vi "tt_timeandsamples.vi"(6 "bin":dbl, 9 "refreshtime":dbl, 10 "srateAODOtt":dbl, 11 "tot#ofsamples":i32) -> (1 "refreshrate":dbl, 2 "refreshbuffer":i32, 3 "timetracecycles":i32)   [LabVIEW 2015]
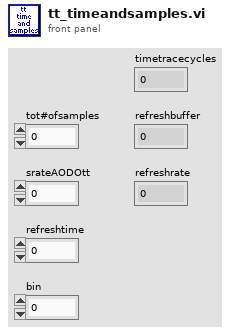
[diagram p1: front panel]
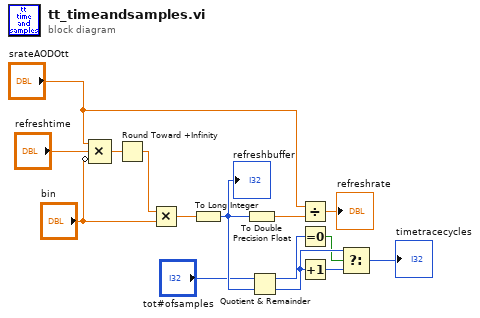
[diagram p0: block diagram]
diagram:
  n1 = Compound Arithmetic op=MULTIPLY("srateAODOtt", "refreshtime", invert "bin") -> (w2:dbl)
  n2 = Round Toward +Infinity(x=w2) -> (ceil(x): smallest int >= x=w9:dbl)
  n3 = Multiply(x=w9, y="bin") -> (x*y=w10:dbl)
  n4 = To Long Integer(number=w10) -> (32bit integer=w12:i32)
  "refreshbuffer" <- w12
  n5 = To Double Precision Float(number=w12) -> (double precision float=w13:dbl)
  n6 = Quotient & Remainder(x="tot#ofsamples", y=w12) -> (x-y*floor(x/y)=w4:i32, floor(x/y)=w7:i32)
  n7 = Divide(x="srateAODOtt", y=w13) -> (x/y=→"refreshrate":dbl)
  n8 = Equal To 0?(x=w4) -> (x = 0?=w5:bool)
  n9 = Increment(x=w7) -> (x+1=w6:i32)
  n10 = Select(t=w7, s=w5, f=w6) -> (s? t:f=→"timetracecycles":i32)
